vi "Lambda2.vi"() -> ()   [LabVIEW 2014]
uses:
  <vilib>/Utility/inputDevices.llb/keyboardAcquire.vi
  <vilib>/Utility/inputDevices.llb/closeKeyboard.vi
  <userlib>/Madlib/Madlib.dll
panel:
  in  "?":string="O / L"
  in  "?":string="D / A"
  in  "?":string="W / S"
  in  "Max Velocity":string(combo)="22"
  in  "Z Decreasing":string(combo)="21"
  in  "Z Increasing":string(combo)="24"
  out "Z Range (mM)":dbl
  out "Y Range (mM)":dbl
  out "X Range (mM)":dbl
  out "Z (mM)":dbl format="%.3f"
  out "Y (mM)":dbl format="%.3f"
  out "X (mM)":dbl format="%.3f"
  in  "X Increasing":string(combo)="32"
  in  "X Decreasing":string(combo)="28"
  in  "Y Decreasing":string(combo)="10"
  in  "Y Increasing":string(combo)="13"
  in  "Motion Multiplier":dbl(slide)=1.0 scale=1.0..100.0
  in  "Command rate":u16(ring)=10 items=["500 Hertz"=2, "100 Hertz"=10, "10 Hertz"=100, "1 Hertz"=1000]
  in  "Camera Shutter":bool
  in  "Wheel Speed":u8=4 min=1 max=7 step=1
  out "Automatic Control":bool=TRUE
  out "Current Filter Wheel Position":string
  in  "Stop Button":bool
  in  "Laser Shutter":T1(radio)
  out "First Key":T2(ring)
  # "l2"
  # "(Lower is faster)"
  # "Nanopositioner"
  # "Command Rate"
  # "Motion Multiplier"
  # "x1"
  # "x100"
  # "Key Configuration"
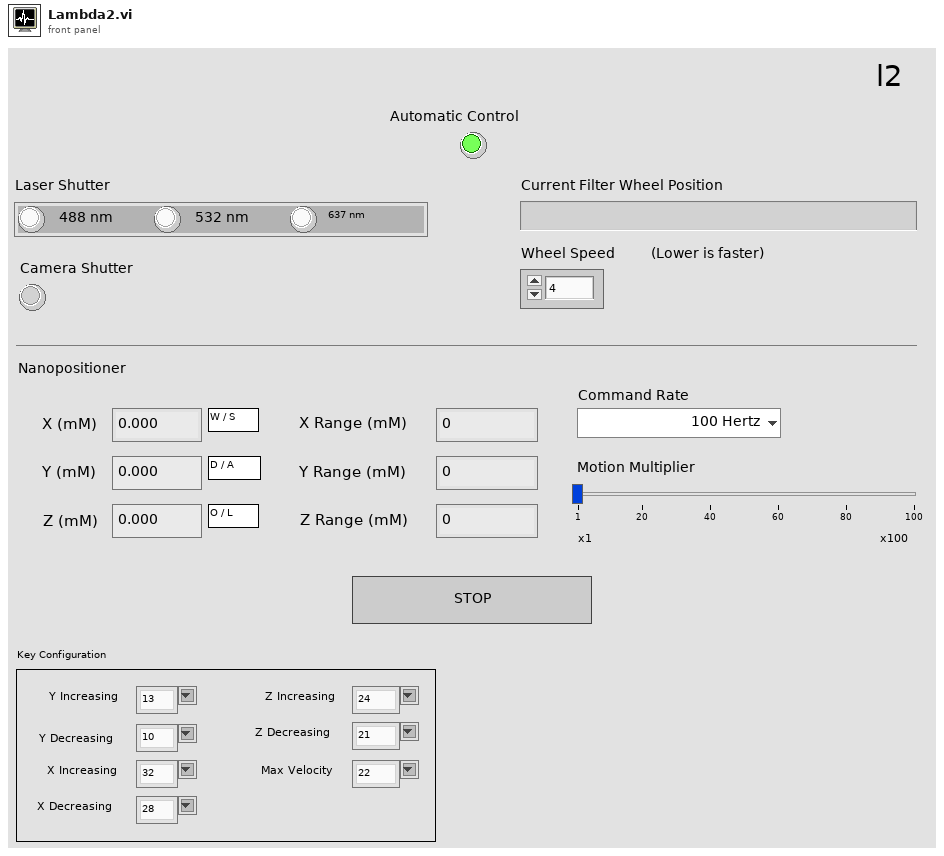
[diagram p1: front panel]
types:
  T1 = enum32{"No Selection", "   488 nm   ", "   532 nm   ", "   637 nm   "}
  T2 = enum16{"0", "1", "2", "3", "4", "5", "6", "7", "8", "9", "A", "B", "C", "D", "E", "F", "G", "H", "I", "J", "K", "L", "M", "N", "O", "P", "Q", "R", "S", "T", "U", "V", "W", "X", "Y", "Z", "F1", "F2", "F3", "F4", "F5", "F6", "F7", "F8", "F9", "F10", "F11", "F12", "F13", "F14", "F15", "ADD", "BACK", "BACKSLASH", "CAPITAL", "COMMA", "DECIMAL", "DELETE", "DIVIDE", "DOWN", "END", "EQUALS", "ESCAPE", "GRAVE (`)", "HOME", "INSERT", "LBRACKET", "LCONTROL", "LEFT", "L ALT", "LSHIFT", "LWIN", "MINUS", "MULTIPLY", "NEXT", "NUMLOCK", "NUMPAD_0", "NUMPAD_1", "NUMPAD_2", "NUMPAD_3", "NUMPAD_4", "NUMPAD_5", "NUMPAD_6", "NUMPAD_7", "NUMPAD_8", "NUMPAD_9", "PAUSE", "PERIOD", "PRIOR (PG UP)", "RBRACKET", "RCONTROL", "RETURN", "RIGHT", "R ALT", "RSHIFT", "RWIN", "SCROLL", "SEMICOLON", "SLASH", "SPACE", "SUBTRACT", "TAB", "UP", "ENTER (num pad)", "' (quote)"}
  T3 = cluster{"X Command":dbl, "Y Command":dbl, "Z Command":dbl, "X Position":dbl, "Y Position":dbl, "Z Position":dbl, "X Calibration":dbl, "Y Calibration":dbl, "Z Calibration":dbl}
  T4 = cluster{"X Command":dbl, "Y Command":dbl, "Z Command":dbl, "X Position":dbl, "Y Position":dbl, "Z Position":dbl}
  T5 = enum16{"0", "1", "2", "3", "4", "5", "6", "7", "8", "9", "A", "B", "C", "D", "E", "F", "G", "H", "I", "J", "K", "L", "M", "N", "O", "P", "Q", "R", "S", "T", "U", "V", "W", "X", "Y", "Z", "F1", "F2", "F3", "F4", "F5", "F6", "F7", "F8", "F9", "F10", "F11", "F12", "F13", "F14", "F15", "ADD", "BACK", "BACKSLASH", "CAPITAL", "COMMA", "DECIMAL", "DELETE", "DIVIDE", "DOWN", "END", "EQUALS", "ESCAPE", "GRAVE (`)", "HOME", "INSERT", "LBRACKET", "LCONTROL", "LEFT", "L ALT", "LSHIFT", "LWIN", "MINUS", "MULTIPLY", "NEXT", "NUMLOCK", "NUMPAD_0", "NUMPAD_1", "NUMPAD_2", "NUMPAD_3", "NUMPAD_4", "NUMPAD_5", "NUMPAD_6", "NUMPAD_7", "NUMPAD_8", "NUMPAD_9", "PAUSE", "PERIOD", "PRIOR (PG UP)", "RBRACKET", "RCONTROL", "RETURN", "RIGHT", "R ALT", "RSHIFT", "RWIN", "SCROLL", "SEMICOLON", "SLASH", "SPACE", "SUBTRACT", "TAB", "UP", "ENTER (num pad)", "' (quote)"}[]
  T6 = cluster{"Y Increasing":string, "Y Decreasing":string, "X Decreasing":string, "X Increasing":string, "Z Increasing":string, "Z Decreasing":string, "Max Velocity":string}
  T7 = cluster{"X Command":dbl, "Y Command":dbl, "Pos. Command":dbl, "X Position":dbl, "Y Position":dbl, "position":dbl}
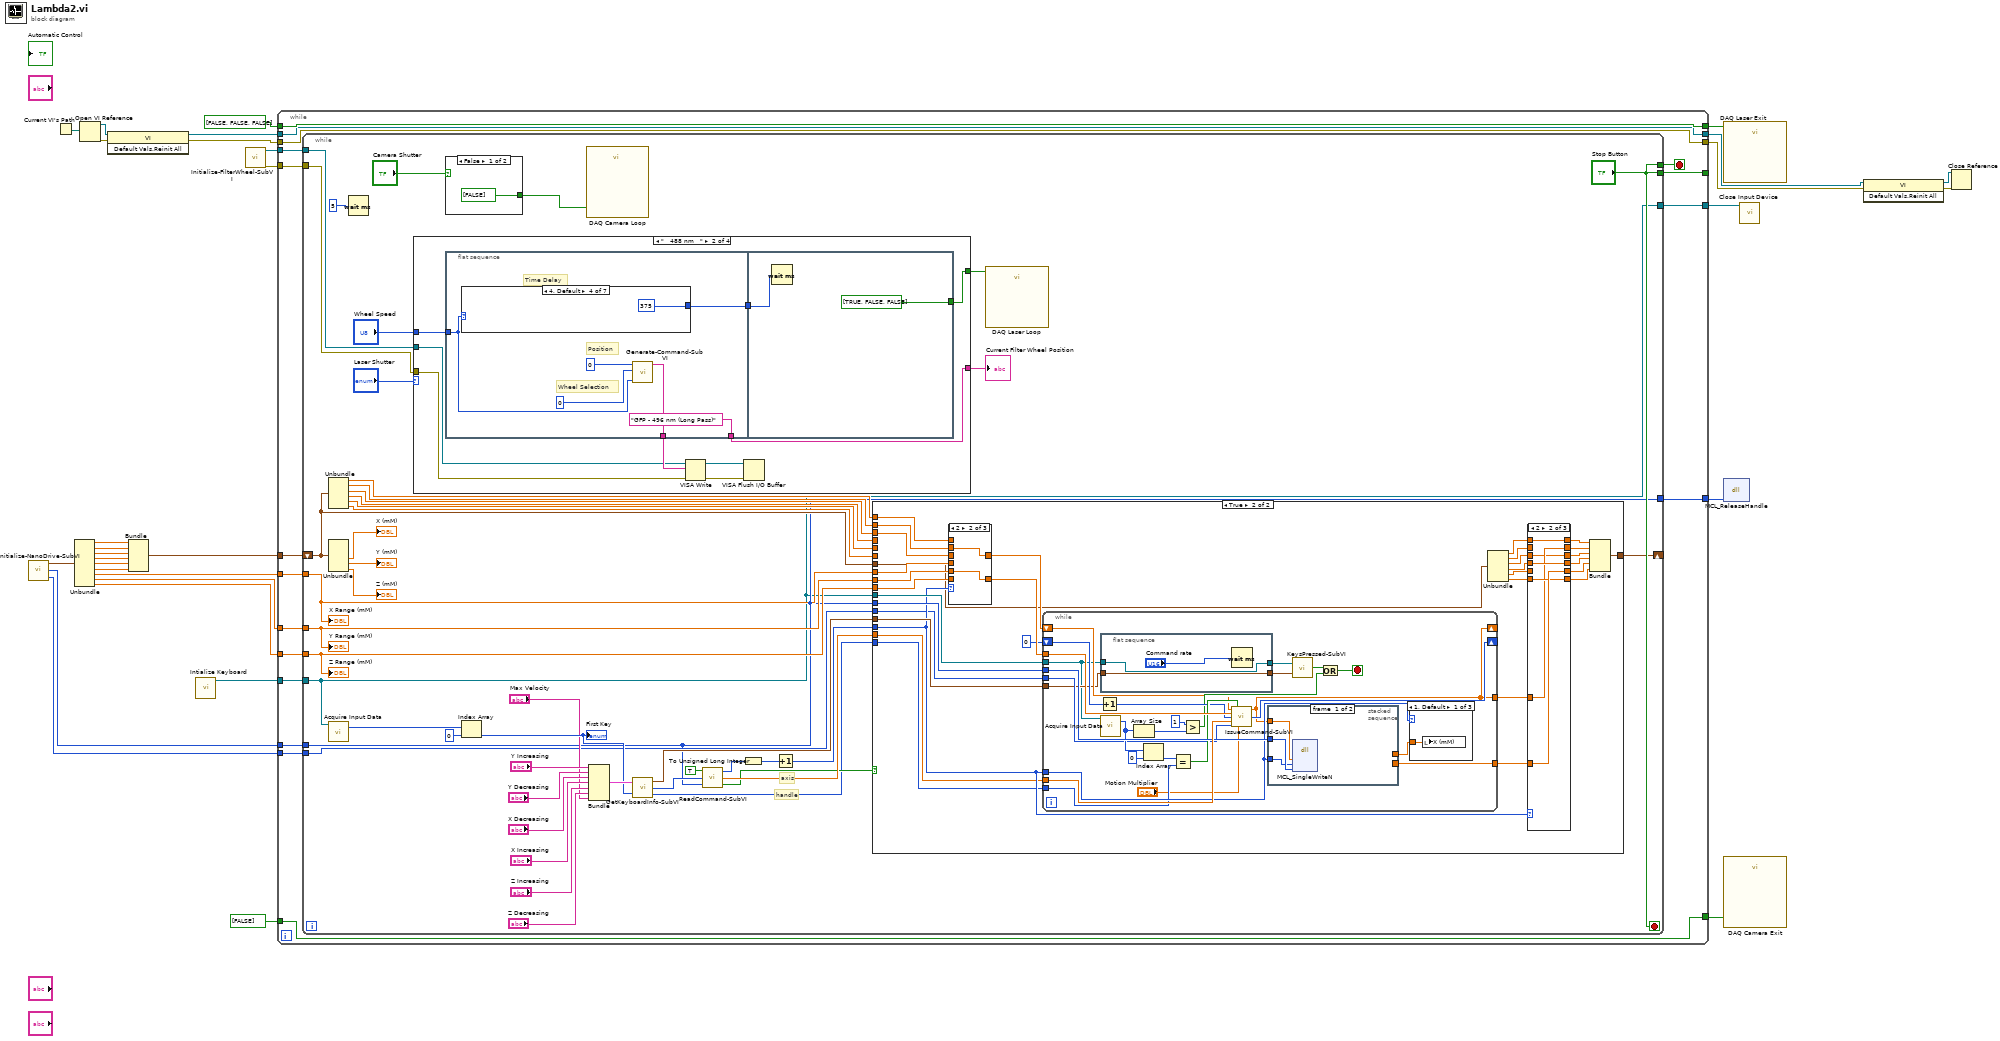
[diagram p0: block diagram]
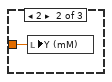
[diagram p7: hidden frame]
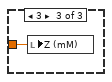
[diagram p8: hidden frame]
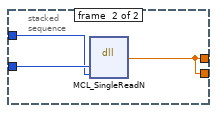
[diagram p9: hidden frame]
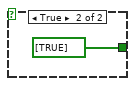
[diagram p10: hidden frame]
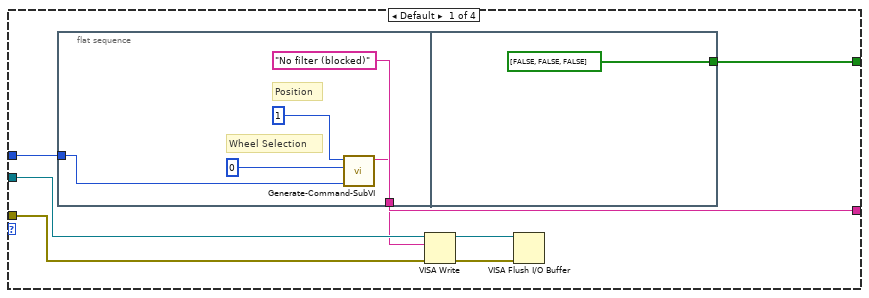
[diagram p11: hidden frame]
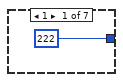
[diagram p12: hidden frame]
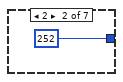
[diagram p13: hidden frame]
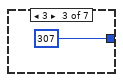
[diagram p14: hidden frame]
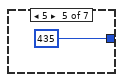
[diagram p15: hidden frame]
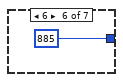
[diagram p16: hidden frame]
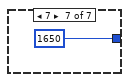
[diagram p17: hidden frame]
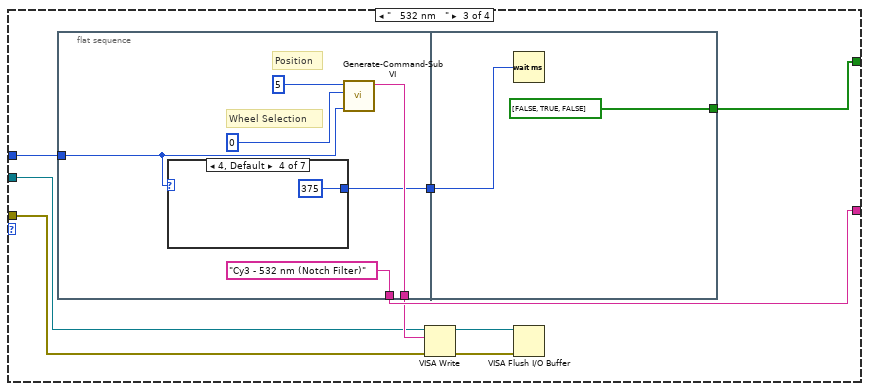
[diagram p18: hidden frame]
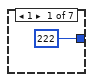
[diagram p19: hidden frame]
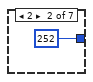
[diagram p20: hidden frame]
diagram:
  n1 = call <userlib>:"Initialize-NanoDrive-SubVI.vi"() -> ("Output Pos Info"=w16:T3, "Handle"=w9:i32, "ADC/DAC Resolution"=w8:u32)  [unwired: 1 out]
  n2 = Current VI's Path() -> (path=w31:path)
  n3 = Unbundle(w16) -> ("X Command"=w15:dbl, "Y Command"=w14:dbl, "Z Command"=w13:dbl, "X Position"=w12:dbl, "Y Position"=w11:dbl, "Z Position"=w10:dbl, "X Calibration"=w6:dbl, "Y Calibration"=w5:dbl, "Z Calibration"=w4:dbl)
  n4 = Open VI Reference(vi path=w31) -> (vi reference=w18:refnum<vi>, error out=w17:errorcluster)  [unwired: 5 in]
  n5 = invoke class="VI" method="Default Vals.Reinit All"(reference=w18, error in=w17) -> (reference out=w20:refnum<vi>, error out=w19:errorcluster)  [unwired: 1 in, 1 out]
  n6 = Bundle("X Command"=w15, "Y Command"=w14, "Z Command"=w13, "X Position"=w12, "Y Position"=w11, "Z Position"=w10) -> (w7:T4)  [unwired: 1 out]
  n7 = call <vilib>:"Intialize Keyboard.vi"() -> ("device ID"=w3:refnum<k1>)  [unwired: 1 in, 10 out]
  n8 = call <userlib>:"Initialize-FilterWheel-SubVI.vi"() -> ("VISA resource name out"=w24:refnum<visa-resource-name>, "error out"=w23:errorcluster)  [unwired: 9 in]
  n9 = while {
    tunnel: [w42] -> w30
    tunnel: [w41] -> w29
    tunnel: bool[] [FALSE, FALSE, FALSE] -> [w47]
    tunnel: [w47] -> w25
    tunnel: w24 -> [w46]
    tunnel: w23 -> [w45]
    tunnel: [w44] -> _
    tunnel: [w43] -> w22
    tunnel: bool[] [FALSE] -> [w43]
    tunnel: w20 -> [w42]
    tunnel: w19 -> [w41]
    tunnel: w9 -> [w40]
    tunnel: w8 -> [w39]
    tunnel: w7 -> [w38]
    tunnel: w6 -> [w37]
    tunnel: w5 -> [w36]
    tunnel: w4 -> [w35]
    tunnel: w3 -> [w34]
    tunnel: [w33] -> w2
    tunnel: [w32] -> w1
    stop <- w48 stop-if-true
    n10 = while {
      tunnel: ["Stop Button"] -> w48
      tunnel: w46 -> [w91]
      tunnel: w45 -> [w90]
      tunnel: ["Stop Button"] -> w44
      tunnel: w40 -> [w50]
      tunnel: w39 -> [w52]
      tunnel: w37 -> [w55]
      tunnel: w36 -> [w54]
      tunnel: w35 -> [w53]
      shift-right: [w51] -> _
      shift-left: w38 -> [w56]
      tunnel: w34 -> [w49]
      tunnel: [w50] -> w33
      tunnel: [w49] -> w32
      stop <- "Stop Button" stop-if-true
      # "handle"
      # "axis"
      n11 = Unbundle(w56) -> ("X Command"=w60:dbl, "Y Command"=w61:dbl, "Z Command"=w62:dbl, "X Position"=w63:dbl, "Y Position"=w64:dbl, "Z Position"=w65:dbl)
      n12 = Unbundle(w56) -> ("X Position"=→"X (mM)":dbl, "Y Position"=→"Y (mM)":dbl, "Z Position"=→"Z (mM)":dbl)  [unwired: 3 out]
      n13 = call-poly <vilib>:"Acquire Input Data.vi"("device ID"=w49) -> ("keys pressed"=w84:T5)  [unwired: 1 in, 17 out]
      n14 = Wait (ms)(milliseconds to wait=5) -> ()  [unwired: 1 out]
      n15 = case shown="\"   488 nm   \"" "Laser Shutter" {
        tunnel: [w201 w216 w240 w263] -> w95
        tunnel: [w200 w215 w239 w264] -> w92
        tunnel: w91 -> [w199 w213 w237 w261]
        tunnel: w90 -> [w198 w212 w236 w260]
        tunnel: "Wheel Speed" -> [w194 w209 w233 w257]
        frame Default {
          n16 = flat-sequence {
            tunnel: [w202] -> w197
            tunnel: ["No filter (blocked)"] -> w200
            tunnel: w194 -> [w203]
            tunnel: [bool[] [FALSE, FALSE, FALSE]] -> w201
            frame #0 {
              # "Wheel Selection"
              # "Position"
              n17 = call <userlib>:"Generate-Command-SubVI.vi"("Wheel Speed"=w203, "Wheel Selection"=u8 0, "Wheel Position"=u8 1) -> ("type"=w202:string)  [unwired: 8 in]
            }
            frame #1 {
            }
          }
          n18 = VISA Write(VISA resource name=w199, write buffer=w197, error in (no error)=w198) -> (VISA resource name out=w196:refnum<visa-resource-name>, error out=w195:errorcluster)  [unwired: 1 out]
          n19 = VISA Flush I/O Buffer(VISA resource name=w196, error in (no error)=w195) -> ()  [unwired: 1 in, 2 out]
        }
        frame "   488 nm   " {
          n20 = flat-sequence {
            tunnel: [w219] -> w214
            tunnel: ["GFP - 496 nm (Long Pass)"] -> w215
            tunnel: w209 -> [w217]
            tunnel: [w218] -> w208
            tunnel: [bool[] [TRUE, FALSE, FALSE]] -> w216
            tunnel: w208 -> [w230]
            frame #0 {
              # "Time Delay"
              # "Wheel Selection"
              # "Position"
              n21 = case shown="4, Default" w217 {
                tunnel: [222 252 307 375 435 885 1650] -> w218
                frame 1 {
                }
                frame 2 {
                }
                frame 3 {
                }
                frame 4, Default {
                }
                frame 5 {
                }
                frame 6 {
                }
                frame 7 {
                }
              }
              n22 = call <userlib>:"Generate-Command-SubVI.vi"("Wheel Speed"=w217, "Wheel Selection"=u8 0, "Wheel Position"=u8 0) -> ("type"=w219:string)  [unwired: 8 in]
            }
            frame #1 {
              n23 = Wait (ms)(milliseconds to wait=w230) -> ()  [unwired: 1 out]
            }
          }
          n24 = VISA Write(VISA resource name=w213, write buffer=w214, error in (no error)=w212) -> (VISA resource name out=w211:refnum<visa-resource-name>, error out=w210:errorcluster)  [unwired: 1 out]
          n25 = VISA Flush I/O Buffer(VISA resource name=w211, error in (no error)=w210) -> ()  [unwired: 1 in, 2 out]
        }
        frame "   532 nm   " {
          n26 = flat-sequence {
            tunnel: ["Cy3 - 532 nm (Notch Filter)"] -> w239
            tunnel: [w243] -> w238
            tunnel: w233 -> [w242]
            tunnel: [w241] -> w232
            tunnel: [bool[] [FALSE, TRUE, FALSE]] -> w240
            tunnel: w232 -> [w254]
            frame #0 {
              # "Wheel Selection"
              # "Position"
              n27 = case shown="4, Default" w242 {
                tunnel: [222 252 307 375 435 885 1650] -> w241
                frame 1 {
                }
                frame 2 {
                }
                frame 3 {
                }
                frame 4, Default {
                }
                frame 5 {
                }
                frame 6 {
                }
                frame 7 {
                }
              }
              n28 = call <userlib>:"Generate-Command-SubVI.vi"("Wheel Speed"=w242, "Wheel Selection"=u8 0, "Wheel Position"=u8 5) -> ("type"=w243:string)  [unwired: 8 in]
            }
            frame #1 {
              n29 = Wait (ms)(milliseconds to wait=w254) -> ()  [unwired: 1 out]
            }
          }
          n30 = VISA Write(VISA resource name=w237, write buffer=w238, error in (no error)=w236) -> (VISA resource name out=w235:refnum<visa-resource-name>, error out=w234:errorcluster)  [unwired: 1 out]
          n31 = VISA Flush I/O Buffer(VISA resource name=w235, error in (no error)=w234) -> ()  [unwired: 1 in, 2 out]
        }
        frame "   637 nm   " {
          n32 = flat-sequence {
            tunnel: ["Cy5 - 637 (Notch Filter)"] -> w264
            tunnel: [w267] -> w262
            tunnel: w257 -> [w266]
            tunnel: [w265] -> w256
            tunnel: [bool[] [FALSE, FALSE, TRUE]] -> w263
            tunnel: w256 -> [w278]
            frame #0 {
              n33 = call <userlib>:"Generate-Command-SubVI.vi"("Wheel Speed"=w266, "Wheel Selection"=u8 0, "Wheel Position"=u8 7) -> ("type"=w267:string)  [unwired: 8 in]
              n34 = case shown="4, Default" w266 {
                tunnel: [222 252 307 375 435 885 1650] -> w265
                frame 1 {
                }
                frame 2 {
                }
                frame 3 {
                }
                frame 4, Default {
                }
                frame 5 {
                }
                frame 6 {
                }
                frame 7 {
                }
              }
            }
            frame #1 {
              n35 = Wait (ms)(milliseconds to wait=w278) -> ()  [unwired: 1 out]
            }
          }
          n36 = VISA Write(VISA resource name=w261, write buffer=w262, error in (no error)=w260) -> (VISA resource name out=w259:refnum<visa-resource-name>, error out=w258:errorcluster)  [unwired: 1 out]
          n37 = VISA Flush I/O Buffer(VISA resource name=w259, error in (no error)=w258) -> ()  [unwired: 1 in, 2 out]
        }
      }
      "Current Filter Wheel Position" <- w92
      n38 = case shown="False" "Camera Shutter" {
        tunnel: [bool[] [FALSE] bool[] [TRUE]] -> w86
        frame False {
        }
        frame True {
        }
      }
      n39 = Index Array "Index Array"(array=w84, index=0) -> (element=w69:T2)
      "First Key" <- w69
      n40 = call "DAQ Camera Loop"("data"=w86) -> ()  [unwired: 17 in, 2 out]
      n41 = Bundle("Y Increasing"="Y Increasing", "Y Decreasing"="Y Decreasing", "X Decreasing"="X Decreasing", "X Increasing"="X Increasing", "Z Increasing"="Z Increasing", "Z Decreasing"="Z Decreasing", "Max Velocity"="Max Velocity") -> (w70:T6)  [unwired: 1 out]
      n42 = call <userlib>:"GetKeyboardInfo-SubVI.vi"("Key Selections"=w70, "Key\nValue"=w69) -> ("Key values"=w81:cluster{i32, i32, i32, i32, i32, i32, i32}, "number"=w83:u32, "Max Velocity Value"=w66:i32)
      n43 = call <userlib>:"ReadCommand-SubVI.vi"("handle"=w50, "Motion #"=w83, "Enable\n(True)"=TRUE ("JoyStick Option")) -> ("Enable Move\n(TRUE)"=w67:bool, "Direction"=w77:dbl, "Axis"=w80:enum16{"X", "Y", "Z"})
      n44 = To Unsigned Long Integer(number=w80) -> (unsigned 32bit integer=w79:u32)
      n45 = Increment(x=w79) -> (x+1=w78:u32)
      n46 = case shown="True" w67 {
        tunnel: w50 -> [_ w128]
        tunnel: w49 -> [_ w127]
        tunnel: w81 -> [_ w126]
        tunnel: w63 -> [_ _]
        tunnel: w64 -> [_ _]
        tunnel: w65 -> [_ _]
        tunnel: w78 -> [_ w124]
        tunnel: w77 -> [_ w122]
        tunnel: w55 -> [_ w121]
        tunnel: w54 -> [_ w120]
        tunnel: w53 -> [_ w119]
        tunnel: w66 -> [_ w116]
        tunnel: w56 -> [w96 w115]
        tunnel: [w96 w114] -> w51
        tunnel: w52 -> [_ w113]
        tunnel: w62 -> [_ w104]
        tunnel: w61 -> [_ w105]
        tunnel: w60 -> [_ w106]
        frame False {
        }
        frame True {
          n47 = case shown="2" w124 {
            tunnel: w106 -> [w148 _ _]
            tunnel: w105 -> [_ w150 _]
            tunnel: w104 -> [_ _ w152]
            tunnel: [w148 w150 w152] -> w125
            tunnel: w121 -> [w147 _ _]
            tunnel: w120 -> [_ w149 _]
            tunnel: w119 -> [_ _ w151]
            tunnel: [w147 w149 w151] -> w118
            frame 1, Default {
            }
            frame 2 {
            }
            frame 3 {
            }
          }
          n48 = while {
            tunnel: w128 -> [w175]
            tunnel: w127 -> [w153]
            tunnel: w126 -> [w155]
            tunnel: w124 -> [w174]
            tunnel: [w178] -> w123
            tunnel: w122 -> [w177]
            tunnel: w118 -> [w176]
            shift-right: [w157] -> _
            shift-left: w125 -> [w158]
            shift-right: [w167] -> _
            shift-left: 0 -> [w169]
            tunnel: w116 -> [w166]
            tunnel: w113 -> [w159]
            tunnel: [w157] -> w103
            stop <- w165 stop-if-true
            n49 = Increment(x=w169) -> (x+1=w168:i32)
            n50 = flat-sequence {
              tunnel: [w181] -> w156
              tunnel: w153 -> [w181]
              tunnel: [w180] -> w154
              tunnel: w155 -> [w180]
              frame #0 {
                n51 = Wait (ms)(milliseconds to wait="Command rate") -> ()  [unwired: 1 out]
              }
            }
            n52 = call-poly <vilib>:"Acquire Input Data.vi"("device ID"=w153) -> ("keys pressed"=w161:T5)  [unwired: 1 in, 17 out]
            n53 = Array Size(array=w161) -> (size(s)=w163:i32)
            n54 = Index Array(array=w161, index=0) -> (element=w172:T2)
            n55 = Equal?(x=w172, y=w166) -> (x = y?=w171:bool)
            n56 = Greater?(x=1, y=w163) -> (0:w164:bool)
            n57 = call <userlib>:"IssueCommand-SubVI.vi"("Current Position"=w158, "Max Velocity?"=w171, "Calibration"=w176, "Loop Iteration"=w168, "Direction"=w177, "ADC/DAC Resolution"=w159, "Motion Multiplier"="Motion Multiplier") -> ("Pos. Command"=w157:dbl, "Loop Iteration Out"=w167:i32)  [unwired: 7 out]
            n58 = stacked-sequence {
              tunnel: w175 -> [w188 w190]
              tunnel: w174 -> [w187 w191]
              tunnel: [_ w189] -> w178
              tunnel: w157 -> [w186 _]
              tunnel: [_ w189] -> w170
              frame #0 {
                n59 = dll-call lib="C:/Program Files (x86)/National Instruments/LabVIEW 2014/user.lib/Madlib/Madlib.dll" fn="MCL_SingleWriteN" label="Madlib.dll\nMCL_SingWriteN"("position"=w186, "axis"=w187, "handle"=w188) -> ()  [unwired: 6 in, 3 out]
              }
              frame #1 {
                n60 = dll-call lib="C:/Program Files (x86)/National Instruments/LabVIEW 2014/user.lib/Madlib/Madlib.dll" fn="MCL_SingleReadN" label="Madlib.dll:\nMCL_SingleReadN"("Axis"=w191, "Handle"=w190) -> ("position"=w189:dbl)  [unwired: 5 in, 2 out]
              }
            }
            n61 = call <userlib>:"KeysPressed-SubVI.vi"("Key values"=w154, "device ID"=w156) -> ("Stop = TRUE"=w179:bool)
            n62 = Or(x=w179, y=w164) -> (x .or. y?=w165:bool)
            n63 = case shown="1, Default" w174 {
              tunnel: w170 -> [w183 w184 w185]
              frame 1, Default {
                n64 = local write "X (mM)"(w183) -> ()
              }
              frame 2 {
                n65 = local write "Y (mM)"(w184) -> ()
              }
              frame 3 {
                n66 = local write "Z (mM)"(w185) -> ()
              }
            }
          }
          n67 = Unbundle(w115) -> ("X Command"=w102:dbl, "Y Command"=w101:dbl, "Z Command"=w100:dbl, "X Position"=w112:dbl, "Y Position"=w111:dbl, "Z Position"=w110:dbl)
          n68 = case shown="2" w124 {
            tunnel: w112 -> [_ w139 w145]
            tunnel: w111 -> [w134 _ w144]
            tunnel: w110 -> [w133 w138 _]
            tunnel: w123 -> [w132 w140 w146]
            tunnel: [w132 w139 w145] -> w107
            tunnel: [w134 w140 w144] -> w108
            tunnel: [w133 w138 w146] -> w109
            tunnel: w103 -> [w131 w137 w141]
            tunnel: w102 -> [_ w136 w143]
            tunnel: w101 -> [w130 _ w142]
            tunnel: w100 -> [w129 w135 _]
            tunnel: [w131 w136 w143] -> w97
            tunnel: [w130 w137 w142] -> w98
            tunnel: [w129 w135 w141] -> w99
            frame 1, Default {
            }
            frame 2 {
            }
            frame 3 {
            }
          }
          n69 = Bundle("X Command"=w97, "Y Command"=w98, "Pos. Command"=w99, "X Position"=w107, "Y Position"=w108, "position"=w109) -> (w114:T7)  [unwired: 1 out]
        }
      }
      n70 = call "DAQ Laser Loop"("data"=w95) -> ()  [unwired: 17 in, 2 out]
      "X Range (mM)" <- w55
      "Y Range (mM)" <- w54
      "Z Range (mM)" <- w53
    }
  }
  n71 = call "DAQ Laser Exit"("data"=w25) -> ()  [unwired: 17 in, 2 out]
  n72 = dll-call lib="C:/Program Files (x86)/National Instruments/LabVIEW 2014/user.lib/Madlib/Madlib.dll" fn="MCL_ReleaseHandle" label="Madlib.dll:\nMCL_ReleaseHandle"("handle"=w2) -> ()  [unwired: 4 in, 3 out]
  n73 = call "DAQ Camera Exit"("data"=w22) -> ()  [unwired: 17 in, 2 out]
  n74 = call-poly <vilib>:"Close Input Device.vi"("device ID"=w1) -> ()  [unwired: 1 in, 9 out]
  n75 = invoke class="VI" method="Default Vals.Reinit All"(reference=w30, error in=w29) -> (reference out=w27:refnum<vi>, error out=w28:errorcluster)  [unwired: 1 in, 1 out]
  n76 = Close Reference(reference=w27, error in (no error)=w28) -> ()  [unwired: 1 out]
